vi "select AOI.vi"(8 "error in (no error)":errorcluster, 11 "Thorcam in":refnum<class "Thorcam.lvclass">) -> (0 "error out":errorcluster, 3 "Thorcam out":refnum<class "Thorcam.lvclass">)   [LabVIEW 2012, in "Thorcam.lvclass"]
uses:
  Thorcam.lvclass
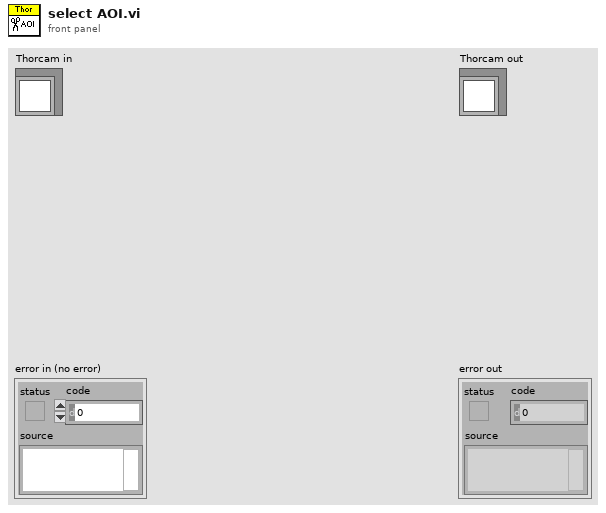
[diagram p1: front panel]
types:
  T1 = typedef "IMAQ Image.ctl" = refnum<image>
  T2 = typedef "ROI Descriptor" = cluster{"Global Rectangle":i32[], "Contours":cluster{"ID":enum32{"External", "Internal"}, "Type":u32, "Coordinates":i32[]}[]}
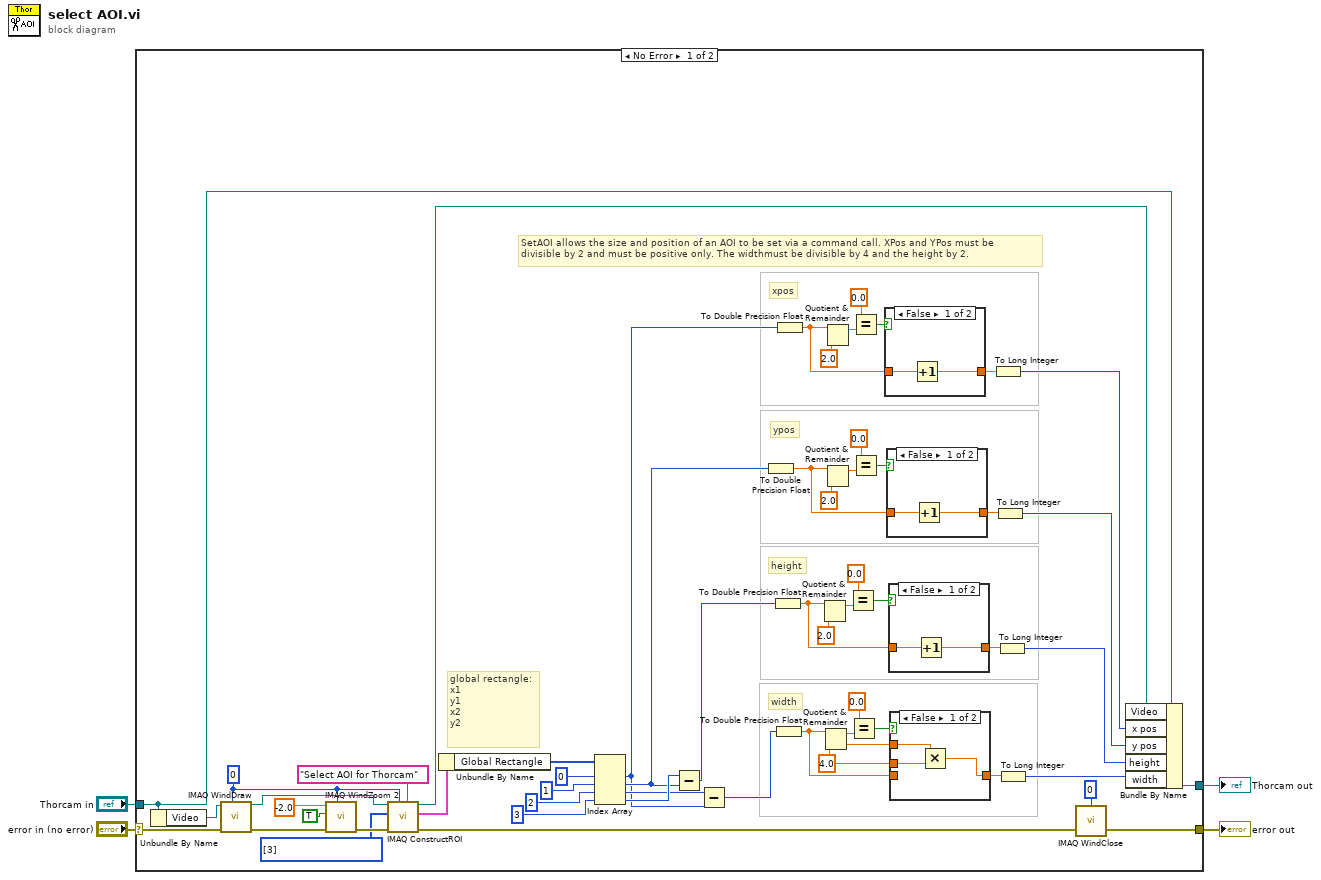
[diagram p0: block diagram]
diagram:
  n1 = case shown="No Error" "error in (no error)" {
    selector: "error in (no error)" -> [w10 w76]
    tunnel: [w6 w76] -> w3
    tunnel: "Thorcam in" -> [w11 w75]
    tunnel: [w48 w75] -> w1
    frame No Error {
      w12 = 4.0 ("y")
      w58 = u32[] [3] items=["No Selection", "Point", "Line", "Rectangle", "Oval", "Polygon", "Freehand Region", "Annulus", "Zoom", "Pan", "Broken Line", "Freehand Line", "Rotated Rectangle"] ("Tools")
      w56 = 0 ("Window Number (0...15)")
      # "global rectangle:\nx1\ny1\nx2\ny2"
      # "SetAOI allows the size and position of an AOI to be set via a command call. XPos and YPos must be\ndivisible by 2 and must be positive only. The widthmust be divisible by 4 and the height by 2."
      # "xpos"
      # "ypos"
      # "height"
      # "width"
      n2 = Unbundle By Name(w11) -> ("Video"=w9:T1)
      n3 = call "IMAQ WindDraw"("Window Number (0...15)"=w56, "error in (no error)"=w10, "Image"=w9) -> ("error out"=w61:errorcluster, "Image Out (duplicate)"=w57:T1)  [unwired: 7 in]
      n4 = call "IMAQ WindZoom 2"("Window Number (0...15)"=w56, "error in (no error)"=w61, "Zoom to Fit? (False)"=TRUE, "Zoom Factor"=sgl -2.0) -> ("error out"=w59:errorcluster)  [unwired: 4 in, 3 out]
      n5 = call "IMAQ ConstructROI"("Prompt"="Select AOI for Thorcam", "Window Number (-1...15)"=w56, "error in (no error)"=w59, "Tools"=w58, "Image"=w57) -> ("error out"=w7:errorcluster, "ROI Descriptor Out"=w54:T2, "Image Out (duplicate)"=w47:T1)  [unwired: 3 in, 1 out]
      n6 = Unbundle By Name(w54) -> ("Global Rectangle"=w53:i32[])
      n7 = Index Array(array=w53, index #1=0 ("index"), index #2=1 ("index"), index #3=2 ("index"), index #4=3 ("index")) -> (element #1=w21:i32, element #2=w25:i32, element #3=w22:i32, element #4=w26:i32)
      n8 = Subtract(x=w26, y=w25) -> (x-y=w24:i32)
      n9 = Subtract(x=w22, y=w21) -> (x-y=w15:i32)
      n10 = To Double Precision Float(number=w25) -> (double precision float=w38:dbl)
      n11 = To Double Precision Float(number=w24) -> (double precision float=w28:dbl)
      n12 = To Double Precision Float(number=w15) -> (double precision float=w19:dbl)
      n13 = To Double Precision Float(number=w21) -> (double precision float=w42:dbl)
      n14 = Quotient & Remainder(x=w28, y=2.0) -> (x-y*floor(x/y)=w31:dbl)  [unwired: 1 out]
      n15 = Quotient & Remainder(x=w19, y=w12) -> (x-y*floor(x/y)=w16:dbl, floor(x/y)=w13:dbl)
      n16 = Quotient & Remainder(x=w42, y=2.0) -> (x-y*floor(x/y)=w45:dbl)  [unwired: 1 out]
      n17 = Quotient & Remainder(x=w38, y=2.0) -> (x-y*floor(x/y)=w35:dbl)  [unwired: 1 out]
      n18 = Equal?(x=0.0, y=w31) -> (x = y?=w29:bool)
      n19 = Equal?(x=0.0, y=w16) -> (x = y?=w18:bool)
      n20 = Equal?(x=0.0, y=w45) -> (x = y?=w43:bool)
      n21 = Equal?(x=0.0, y=w35) -> (x = y?=w37:bool)
      n22 = case shown="False" w43 {
        tunnel: w42 -> [w73 w74]
        tunnel: [w72 w74] -> w41
        frame False {
          n23 = Increment(x=w73) -> (x+1=w72:dbl)
        }
        frame True {
        }
      }
      n24 = case shown="False" w37 {
        tunnel: w38 -> [w70 w71]
        tunnel: [w69 w71] -> w39
        frame False {
          n25 = Increment(x=w70) -> (x+1=w69:dbl)
        }
        frame True {
        }
      }
      n26 = case shown="False" w29 {
        tunnel: w28 -> [w67 w68]
        tunnel: [w66 w68] -> w27
        frame False {
          n27 = Increment(x=w67) -> (x+1=w66:dbl)
        }
        frame True {
        }
      }
      n28 = case shown="False" w18 {
        tunnel: w19 -> [_ w65]
        tunnel: [w64 w65] -> w20
        tunnel: w13 -> [w63 _]
        tunnel: w12 -> [w62 _]
        frame False {
          n29 = Multiply(x=w63, y=w62) -> (x*y=w64:dbl)
        }
        frame True {
        }
      }
      n30 = To Long Integer(number=w41) -> (32bit integer=w40:i32)
      n31 = To Long Integer(number=w39) -> (32bit integer=w33:i32)
      n32 = To Long Integer(number=w27) -> (32bit integer=w23:i32)
      n33 = To Long Integer(number=w20) -> (32bit integer=w14:i32)
      n34 = call "IMAQ WindClose"("Window Number (0...15)"=0, "error in (no error)"=w7) -> ("error out"=w6:errorcluster)  [unwired: 4 in]
      n35 = Bundle By Name(cluster=w11, "Video"=w47, "x pos"=w40, "y pos"=w33, "height"=w23, "width"=w14) -> (w48:refnum<class "Thorcam.lvclass">)
    }
    frame Error {
    }
  }
  "error out" <- w3
  "Thorcam out" <- w1
